vi "Find New Resource.vi"(10 "Previous Resources":refnum<class "VisaResource.lvclass">[](array[class]), 11 "Current Resources":refnum<class "VisaResource.lvclass">[](array[class])) -> (2 "Valid?":bool, 3 "New Resource":refnum<class "VisaResource.lvclass">)   [LabVIEW 2020, in "RP2040.lvlib" / "RP2040Platform.lvclass"]
uses:
  RP2040Platform.lvclass
  Builds/picoG/ppl/PicoG-Core.lvlibp/PicoG-Processor/PicoG-Core/VisaResource/VisaResource.lvclass
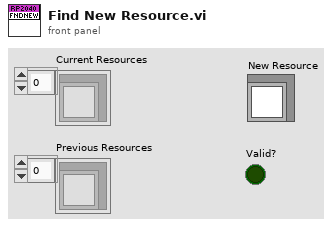
[diagram p1: front panel]
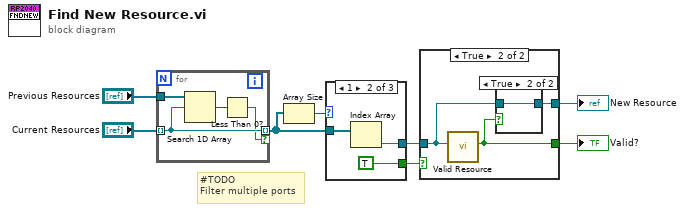
[diagram p0: block diagram]
diagram:
  # "#TODO\nFilter multiple ports"
  n1 = for {
    tunnel: "Current Resources" -> [w10] mode=indexing
    tunnel: "Previous Resources" -> [w12]
    tunnel: [w10] -> w5 mode=indexing if=w9
    n2 = Search 1D Array(1D array=w12, element=w10) -> (index of element=w11:i32)  [unwired: 1 in]
    n3 = Less Than 0?(x=w11) -> (x < 0?=w9:bool)
  }
  n4 = Array Size(array=w5) -> (size(s)=w6:i32)
  n5 = case shown="1" w6 {
    tunnel: w5 -> [_ w15 _]
    tunnel: [_ w14 _] -> w4
    tunnel: [_ TRUE _] -> w3
    frame 0 {
    }
    frame 1 {
      n6 = Index Array(array=w15) -> (element=w14:refnum<class "VisaResource.lvclass">)  [unwired: 1 in]
    }
    frame Default {
    }
  }
  n7 = case shown="True" w3 {
    tunnel: w4 -> [_ w17]
    tunnel: [_ w18] -> w2
    tunnel: [_ w16] -> w1
    frame False {
    }
    frame True {
      n8 = call "Valid Resource.vi"("RP2040.lvlib:VisaResource"=w17) -> ("Valid?"=w18:bool)  [unwired: 9 in, 1 out]
      n9 = case shown="True" w18 {
        tunnel: w17 -> [_ w19]
        tunnel: [_ w19] -> w16
        frame False {
        }
        frame True {
        }
      }
    }
  }
  "New Resource" <- w1
  "Valid?" <- w2
